vi "MSGR Get Q.vi"(8 "error in (no error)":errorcluster, 11 "MSGR Q name":T3) -> (0 "error out":errorcluster, 3 "MSGR Q":T1)   [LabVIEW 2018]
doc: "$Author::Richard Jennings $\n$Rev:: $\n$Date:: May, 2008 $\n\nOVERVIEW:\nReentrant VI to receive messages via a MSGR Q. If the Q does not exist this VI will create it, then wait for data.\n\nINPUTS (Controls):\n<name> - <short description of each control wired to connector pane>\n\nOUTPUTS (Indicators):\n<name> - <short description of each indicator wired to connector pane>\n\nCopyright 2008 - 2017 Jennings Embedded Servies. All rights reserved.\nAuthor makes no warranties or guarantees related to performance of the software.\nUSE AT YOUR OWN RISK\nwww.jembedded.com"
uses:
  MSGR Q Name TypeDef.ctl
  MSGR Q Data TypeDef.ctl
  MSGR Q Ref TypeDef.ctl
  MSGR Registry Control TypeDef.ctl
panel:
  in  "MSGR Q Data TypeDef":T2
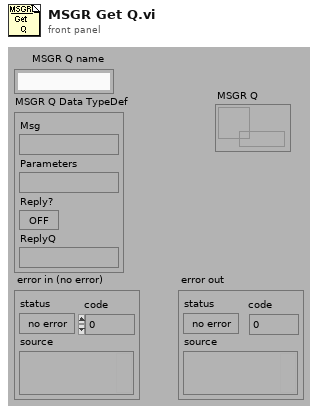
[diagram p1: front panel]
types:
  T1 = typedef "MSGR Q Ref TypeDef.ctl" = refnum<queue>
  T2 = typedef "MSGR Q Data TypeDef.ctl" = cluster{"Msg":string, "Parameters":string, "Reply?":bool, "ReplyQ":string}
  T3 = typedef "MSGR Q Name TypeDef.ctl" = string
  T4 = typedef "MSGR Registry Control TypeDef.ctl" = enum16{"reset", "register", "get data", "set data", "unregister", "test", "get objects"}
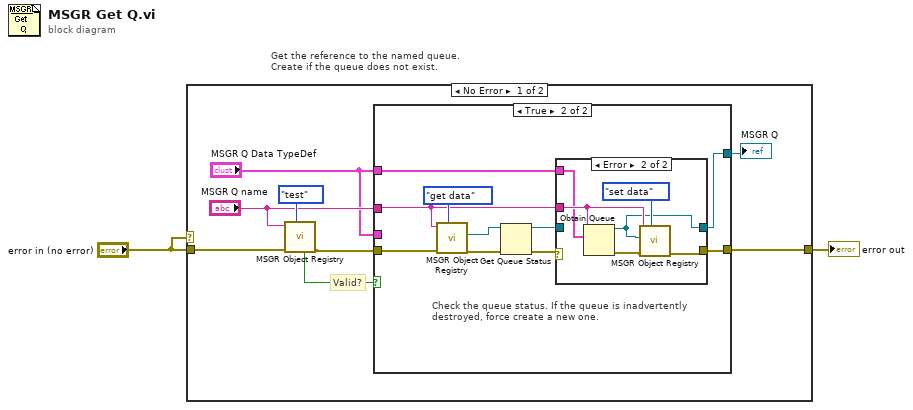
[diagram p0: block diagram]
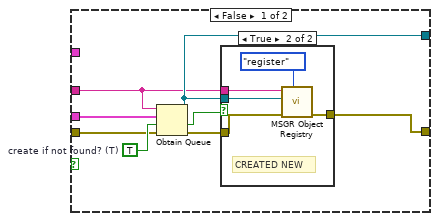
[diagram p2: hidden frame]
diagram:
  # "Get the reference to the named queue.\nCreate if the queue does not exist."
  n1 = case shown="No Error" "error in (no error)" {
    tunnel: [w10 w43] -> w2
    tunnel: "error in (no error)" -> [w7 w43]
    frame No Error {
      # "Valid?"
      n2 = call "MSGR Object Registry.vi"("function (get data)"=MSGR_Registry_Control_TypeDef."test", "error in (no error)"=w7, "MSGR Q name"="MSGR Q name") -> ("error out"=w8:errorcluster, "valid index?"=w6:bool)  [unwired: 1 in, 6 out]
      n3 = case shown="True" w6 {
        tunnel: [w18 w27] -> w10
        tunnel: [w17 w29] -> w9
        tunnel: "MSGR Q Data TypeDef" -> [w14 _]
        tunnel: w8 -> [w12 w34]
        tunnel: "MSGR Q name" -> [w11 w26]
        tunnel: "MSGR Q Data TypeDef" -> [_ w25]
        frame False {
          w15 = TRUE  # create if not found? (T)
          n4 = Obtain Queue(name (unnamed)=w11, element data type=w14, create if not found? (T)=w15, error in (no error)=w12) -> (queue out=w17:refnum<queue>, created new?=w13:bool, error out=w16:errorcluster)  [unwired: 1 in]
          n5 = case shown="True" w13 {
            tunnel: [w19 w24] -> w18
            tunnel: w11 -> [_ w23]
            tunnel: w17 -> [_ w22]
            tunnel: w16 -> [w19 w20]
            frame False {
            }
            frame True {
              # "CREATED NEW"
              n6 = call "MSGR Object Registry.vi"("function (get data)"=MSGR_Registry_Control_TypeDef."register", "error in (no error)"=w20, "MSGR Q"=w22, "MSGR Q name"=w23) -> ("error out"=w24:errorcluster)  [unwired: 7 out]
            }
          }
        }
        frame True {
          # "Check the queue status. If the queue is inadvertently destroyed, force create a new one."
          n7 = call "MSGR Object Registry.vi"("function (get data)"=MSGR_Registry_Control_TypeDef."get data", "error in (no error)"=w34, "MSGR Q name"=w26) -> ("error out"=w32:errorcluster, "MSGR Q"=w31:T1)  [unwired: 1 in, 6 out]
          n8 = Get Queue Status(queue=w31, error in (no error)=w32) -> (queue out=w28:T1, error out=w30:errorcluster)  [unwired: 1 in, 6 out]
          n9 = case shown="Error" w30 {
            selector: w30 -> [w35 _]
            tunnel: [w36 w37] -> w29
            tunnel: w28 -> [w36 _]
            tunnel: [w35 w38] -> w27
            tunnel: w26 -> [_ w42]
            tunnel: w25 -> [_ w41]
            frame No Error {
            }
            frame Error {
              n10 = Obtain Queue(name (unnamed)=w42, element data type=w41) -> (queue out=w37:refnum<queue>, error out=w40:errorcluster)  [unwired: 3 in, 1 out]
              n11 = call "MSGR Object Registry.vi"("function (get data)"=MSGR_Registry_Control_TypeDef."set data", "error in (no error)"=w40, "MSGR Q"=w37, "MSGR Q name"=w42) -> ("error out"=w38:errorcluster)  [unwired: 7 out]
            }
          }
        }
      }
      "MSGR Q" <- w9
    }
    frame Error {
    }
  }
  "error out" <- w2
